vi "_ConnectorPaneEditor_ReadControlsData.vi"(8 "error in (no error)":errorcluster, 11 "ConnectorPaneEditor in":refnum<class "_ConnectorPaneEditor.lvclass">) -> (0 "error out":errorcluster, 1 "TunelsInformation":string[][](array[string]), 2 "RowHeader":string[](array[string]), 3 "ConnectorPaneEditor out":refnum<class "_ConnectorPaneEditor.lvclass">)   [LabVIEW 2014, in "_ConnectorPaneEditor.lvclass"]
uses:
  _ConnectorPaneEditor.lvclass
  _ConnectorPaneEditor.lvclass/_ConnectorPaneEditor.ctl
  <vilib>/Utility/VariantDataType/VariantType.lvlib
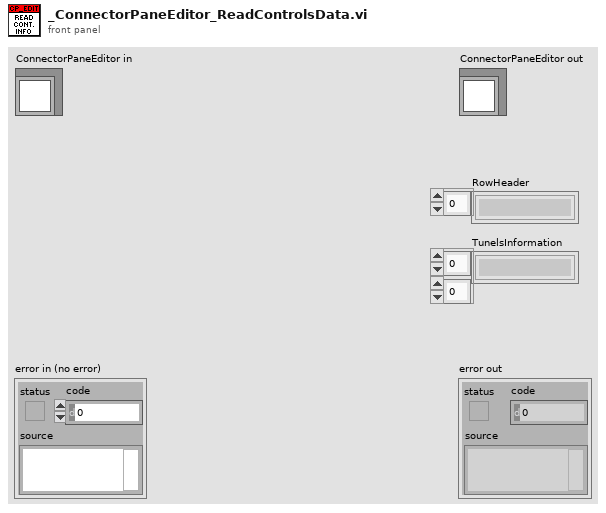
[diagram p1: front panel]
types:
  T1 = enum16{"Invalid Wire Rule", "Required", "Recommended", "Optional", "Dynamic Dispatch"}[]
  T2 = typedef "VariantType.lvlib/Type.ctl" = enum8{"Invalid Type", "Void", "I8", "I16", "I32", "I64", "U8", "U16", "U32", "U64", "Single Float", "Double Float", "Extended Float", "Single Complex", "Double Complex", "Extended Complex", "Enum U8", "Enum U16", "Enum U32", "Enum U64", "Single Float With Unit", "Double Float With Unit", "Extended Float With Unit", "Single Complex with Unit", "Double Complex with Unit", "Extended Complex with Unit", "Boolean", "String", "Path", "Picture", "Tag", "Array", "Cluster", "Variant", "LV Variant", "Waveform", "Timestamp", "Digital Waveform", "Digital Data", "ExpressData", "Refnum", "External Data", "VI", "Poly VI", "LabVIEW Class Instance", "Fixed Point"}
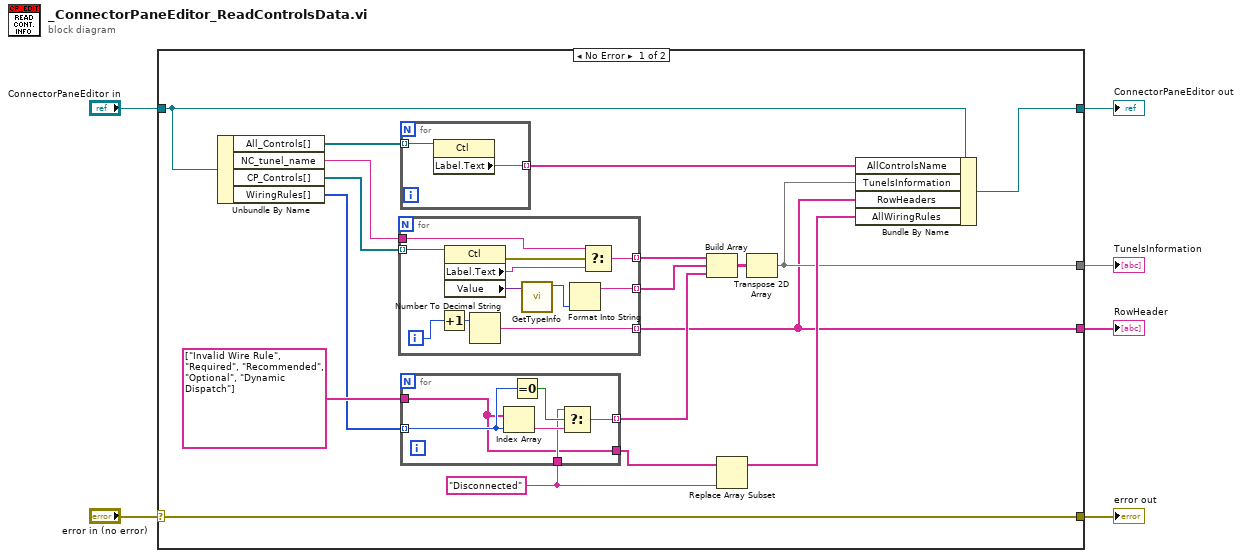
[diagram p0: block diagram]
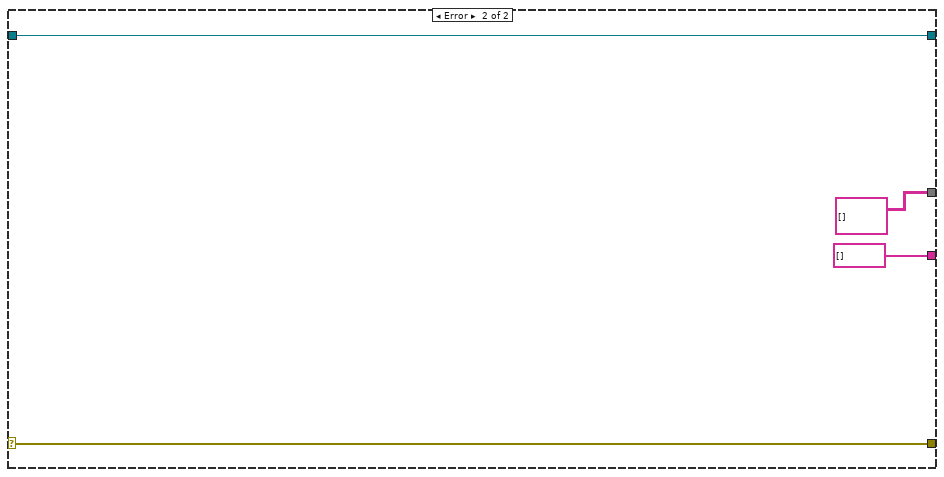
[diagram p2: hidden frame]
diagram:
  n1 = case shown="No Error" "error in (no error)" {
    selector: "error in (no error)" -> [w9 w47]
    tunnel: [w9 w47] -> w5
    tunnel: [w15 w46] -> w3
    tunnel: "ConnectorPaneEditor in" -> [w16 w46]
    tunnel: [w11 string[][] []] -> w2
    tunnel: [w10 string[] []] -> w1
    frame No Error {
      w24 = "Disconnected" ("t")
      n2 = Unbundle By Name(w16) -> ("All_Controls[]"=w14:refnum<vi>[], "NC_tunel_name"=w13:string, "CP_Controls[]"=w7:refnum<vi>[], "WiringRules[]"=w8:T1)
      n3 = for {
        tunnel: [w34] -> w19 mode=indexing
        tunnel: [w31] -> w10 mode=indexing
        tunnel: [w25] -> w20 mode=indexing
        tunnel: w7 -> [w29] mode=indexing
        tunnel: w13 -> [w30]
        i -> [w33]
        n4 = Increment(x=w33) -> (x+1=w32:i32)
        n5 = property class="Ctl"(reference=w29) -> (error out=w28:errorcluster, "Label.Text"=w35:string, "Value"=w27:variant)  [unwired: 1 in, 1 out]
        n6 = Number To Decimal String(number=w32) -> (decimal integer string=w31:string)  [unwired: 1 in]
        n7 = call <vilib>:"GetTypeInfo.vi"("Variant"=w27) -> ("Type Enum"=w26:T2)  [unwired: 6 in, 4 out]
        n8 = Format Into String(w26) -> (resulting string=w25:string)  [unwired: 3 in, 1 out]
        n9 = Select(t=w30, s=w28, f=w35) -> (s? t:f=w34:string)
      }
      n10 = for {
        tunnel: w14 -> [w37] mode=indexing
        tunnel: [w36] -> w17 mode=indexing
        n11 = property class="Ctl"(reference=w37) -> ("Label.Text"=w36:string)  [unwired: 1 in, 2 out]
      }
      n12 = for {
        tunnel: w8 -> [w41] mode=indexing
        tunnel: [w42] -> w18 mode=indexing
        tunnel: [w38] -> w23
        tunnel: w24 -> [w39]
        tunnel: string[] ["Invalid Wire Rule", "Required", "Recommended", "Optional", "Dynamic Dispatch"] ("Strings [] 2") -> [w38]
        n13 = Index Array(array=w38, index=w41) -> (element=w43:string)
        n14 = Equal To 0?(x=w41) -> (x = 0?=w40:bool)
        n15 = Select(t=w39, s=w40, f=w43) -> (s? t:f=w42:string)
      }
      n16 = Build Array(w19, w20, w18) -> (w21:string[][])
      n17 = Replace Array Subset(array=w23, new element=w24) -> (w22:string[])  [unwired: 1 in]
      n18 = Transpose 2D Array(2D array=w21) -> (transposed array=w11:string[][])
      n19 = Bundle By Name(cluster=w16, "AllControlsName"=w17, "TunelsInformation"=w11, "RowHeaders"=w10, "AllWiringRules"=w22) -> (w15:refnum<class "_ConnectorPaneEditor.lvclass">)
    }
    frame Error {
    }
  }
  "error out" <- w5
  "ConnectorPaneEditor out" <- w3
  "TunelsInformation" <- w2
  "RowHeader" <- w1
